vi "pack_for_storage.vi"(8 "error in":errorcluster, 10 "Data in":T1) -> (0 "error out":errorcluster, 2 "String out":string)   [LabVIEW 2010]
uses:
  typedefs/data_cluster.ctl
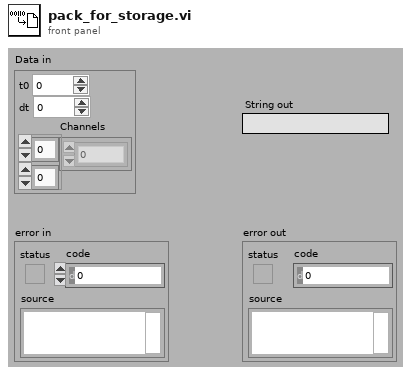
[diagram p1: front panel]
types:
  T1 = typedef "data_cluster.ctl" = cluster{"t0":dbl, "dt":dbl, "Channels":dbl[][]}
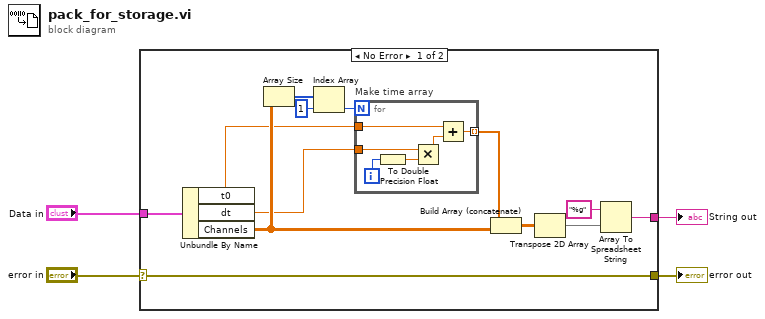
[diagram p0: block diagram]
diagram:
  n1 = case shown="No Error" "error in" {
    selector: "error in" -> [w13 w24]
    tunnel: "Data in" -> [w14 _]
    tunnel: [w15 _] -> w4
    tunnel: [w13 w24] -> w2
    frame No Error {
      n2 = Unbundle By Name(w14) -> ("t0"=w9:dbl, "dt"=w8:dbl, "Channels"=w12:dbl[][])
      n3 = Array Size(array=w12) -> (size(s)=w11:i32[])
      n4 = Index Array(array=w11, index=1) -> (element=w7:i32)
      n5 = for "Make time array" {
        N: w7 -> [_]
        tunnel: w9 -> [w19]
        tunnel: w8 -> [w23]
        tunnel: [w18] -> w6 mode=indexing
        i -> [w21]
        n6 = To Double Precision Float(number=w21) -> (double precision float=w22:dbl)
        n7 = Multiply(x=w23, y=w22) -> (x*y=w20:dbl)
        n8 = Add(x=w19, y=w20) -> (x+y=w18:dbl)
      }
      n9 = Build Array (concatenate)(w6, w12) -> (w5:dbl[][])
      n10 = Transpose 2D Array(2D array=w5) -> (transposed array=w16:dbl[][])
      n11 = Array To Spreadsheet String(array=w16, 3:"%g" ("format string")) -> (spreadsheet string=w15:string)  [unwired: 1 in]
    }
    frame Error {
    }
  }
  "String out" <- w4
  "error out" <- w2
